vi "End Array.vi"   [LabVIEW 2017, in "LabPack.lvlib" / "Writer.lvclass"]
doc: "Finishes writing and encoding an array to the MessagePack binary data format. This VI must be called after writing and encoding all of the array's elements to avoid subsequent errors."
uses:
  Writer.lvclass
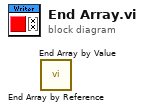
[diagram p0: block diagram]
diagram:
  n1 = call "End Array by Reference.vi"() -> ()  [unwired: 10 in, 2 out]
  n2 = call "End Array by Value.vi"() -> ()  [unwired: 10 in, 2 out]
